vi "main_VI.vi"() -> ()   [LabVIEW 2019]
uses:
  <vilib>/myRIO/Instrument Drivers/Onboard IO/UART/typedef/VISA Configuration.ctl
  <vilib>/Platform/TimedLoop/XDataNode/timing_clust.ctl
  <vilib>/Platform/TimedLoop/XDataNode/nitl_modes.ctl
  <vilib>/Platform/TimedLoop/XDataNode/wakeup.ctl
  <vilib>/myRIO/Instrument Drivers/Onboard IO/AI/typedefs/AI Reference.ctl
  <vilib>/myRIO/Common/Instrument Driver Framework/Utilities/typedefs/myRIO Generic Hardware Reference.ctl
  <vilib>/myRIO/Common/Instrument Driver Framework/Utilities/typedefs/Hardware Version Enum.ctl
  <vilib>/myRIO/Common/Instrument Driver Framework/Utilities/typedefs/myRIO v1.0 Reference.ctl
  <vilib>/myRIO/Common/Instrument Driver Framework/Utilities/typedefs/Generic FPGA Reference.ctl
  <vilib>/myRIO/Common/Instrument Driver Framework/myRIO v1.0/AI/typedefs/AI Channels List.ctl
  <vilib>/myRIO/Common/Instrument Driver Framework/myRIO v1.0/AI/typedefs/AI Channels Enum.ctl
  <vilib>/myRIO/Common/Instrument Driver Framework/Utilities/typedefs/Analog Scaling Constants List.ctl
  <vilib>/myRIO/Common/Instrument Driver Framework/Utilities/typedefs/Analog Scaling Constants.ctl
  <vilib>/userDefined/High Color/nirio_resource_hc.ctl
  <vilib>/Instr/_visa.llb/VISA Configure Serial Port (Instr).vi
  <vilib>/myRIO/Instrument Drivers/Onboard IO/AI/vis/Read.vi
  <vilib>/myRIO/Common/Instrument Driver Framework/myRIO v1.0/AI/vis/myRIO v1.1 Open AI.vi
  <vilib>/myRIO/Common/Instrument Driver Framework/Utilities/vis/Is FPGA Ref Available.vi
  <vilib>/myRIO/Common/Instrument Driver Framework/Utilities/vis/Validate Channels.vi
  <vilib>/myRIO/Common/Instrument Driver Framework/myRIO v1.0/AI/vis/myRIO v1.0 Reserve AI.vi
  <vilib>/myRIO/Common/Instrument Driver Framework/myRIO v1.0/AI/vis/myRIO v1.0 Build MUX Configuration AI.vi
  <vilib>/myRIO/Common/Instrument Driver Framework/myRIO v1.0/Resource Manager/vis/myRIO v1.0 Reserve Channel List.vi
  <vilib>/myRIO/Common/Instrument Driver Framework/myRIO v1.0/Resource Manager/vis/myRIO v1.0 Reserve Channel.vi
  <vilib>/myRIO/Common/Instrument Driver Framework/myRIO v1.0/Resource Manager/vis/myRIO v1.0 Unreserve Channel.vi
  <vilib>/myRIO/Common/Instrument Driver Framework/myRIO v1.0/Resource Manager/vis/myRIO v1.0 Build Mutex Name.vi
  <vilib>/Utility/VariantDataType/GetNumericInfo.vi
  <vilib>/Utility/error.llb/Error Cluster From Error Code.vi
  <vilib>/myRIO/Common/Instrument Driver Framework/myRIO v1.0/myRIO v1.1 Open.vi
  <vilib>/myRIO/Common/Instrument Driver Framework/myRIO v1.0/AI/vis/myRIO v1.0 Get Scaling Constants AI.vi
  <vilib>/myRIO/Common/Instrument Driver Framework/Utilities/vis/IO Manager.vi
  <vilib>/myRIO/Common/Instrument Driver Framework/Utilities/vis/Configuration Manager.vi
  <vilib>/myRIO/Common/Instrument Driver Framework/myRIO v1.0/myRIO v1.0 Close.vi
  <vilib>/myRIO/Common/Instrument Driver Framework/myRIO v1.0/AI/vis/myRIO v1.0 Read AI.vi
  <vilib>/Utility/file.llb/Write Delimited Spreadsheet (DBL).vi
  <vilib>/platform/TimedLoop/XDataNode/XDataNode.xnode
  <vilib>/myRIO/Express VI/Onboard IO/AI/AI Express VI.xnode
  <vilib>/myRIO/Instrument Drivers/Onboard IO/AI/vis/myRIO AI Open.xnode
  <vilib>/Platform/TimedLoop/XDataNode/XDNodeRunTimeDep.lvlib
  <vilib>/myRIO/Instrument Drivers/Onboard IO/UART/UART.lvlib
  <vilib>/myRIO/Instrument Drivers/Onboard IO/AI/AI.lvlib
panel:
  out "# elements 2":u32
  out "element out 2":dbl
  out "# elements":u32
  out "element out":dbl
  out "Gyro_z":dbl
  in  "error in (no error)":errorcluster
  out "On time in":i32
  out "Late in":i32
  out "Loop cycle rate":u32
  in  "File_Num.":i16
  in  "stop":bool
  out "error out":errorcluster
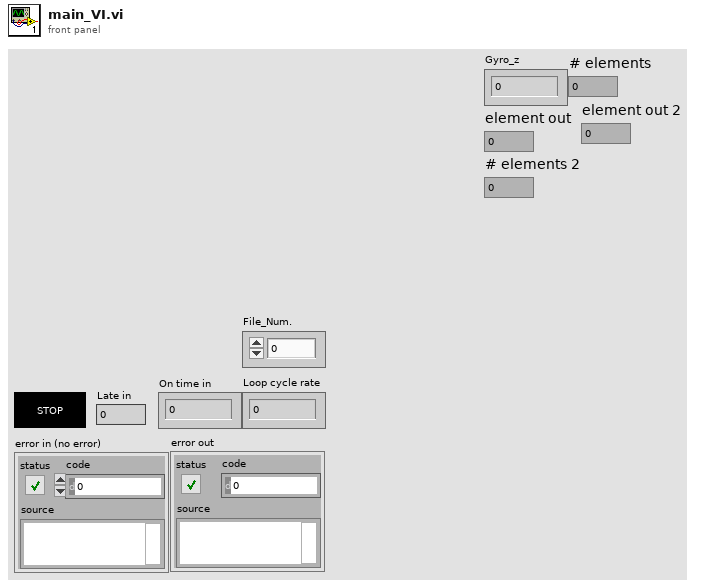
[diagram p1: front panel]
types:
  T1 = cluster{"read mode":enum16{"polling", "blocking"}, "write mode":enum16{"polling", "blocking"}}
  T2 = typedef "UART.lvlib/VISA Configuration.ctl" = cluster{"baud rate (9600)":u32, "data bits (8)":u16, "parity (0:none)":enum16{"None", "Odd", "Even", "Mark", "Space"}, "stop bits (10: 1 bit)":u16, "flow control (0:none)":u16, "termination char\n(0xA = '\\n' = LF) ":u8, "Enable Termination\nChar (T)":bool, "timeout (10sec)":u32}
  T3 = typedef "XDNodeRunTimeDep.lvlib/timing_clust.ctl" = cluster{"Expected End [f-1]":u64, "Actual End [f-1]":u64, "Finished Late? [f-1]":bool, "Expected End [i-1]":u64, "Actual End [i-1]":u64, "Finished Late? [i-1]":bool, "Expected Start [i]":u64, "Actual Start [i]":u64, "Expected Start [f]":u64, "Actual Start [f]":u64, "Source Name":string, "Structure Name":string, "Period":i64, "Deadline":i64, "Offset":i64, "Start":i64, "Priority":i32, "Timeout":i32, "Mode":T4, "Wakeup Reason":T5, "Error":errorcluster, "Source Type":string, "Secondary Source Type":string, "Global End Time":u64, "Global Start Time":u64, "Frame Duration":u64, "Iteration Duration":u64, "Assigned CPU":i32, "I/O Scan Engine Mode":u32}
  T4 = typedef "XDNodeRunTimeDep.lvlib/nitl_modes.ctl" = enum32{"No Change", "Process missed periods, maintain original phase", "Discard missed periods, maintain original phase", "Process missed periods, ignore original phase", "Discard missed periods, ignore original phase"}
  T5 = typedef "XDNodeRunTimeDep.lvlib/wakeup.ctl" = enum32{"Normal", "Aborted", "Asynchronous wakeup", "Timing source error", "Timed loop error", "Timeout"}
  T6 = typedef "AI.lvlib/AI Reference.ctl" = cluster{"myRIO Reference":T7, "AI Channels List":T11, "AI Scaling Constants List":T13}
  T7 = typedef "myRIO Generic Hardware Reference.ctl" = cluster{"myRIO Model":T8, "myRIO Hardware Reference":T9}
  T8 = typedef "Hardware Version Enum.ctl" = enum16{"Unknown", "myRIO-1900", "myRIO-1950", "roboRIO", "NI ELVIS RIO CM", "ELVIS III"}
  T9 = typedef "myRIO v1.0 Reference.ctl" = cluster{"Generic FPGA Reference":T10, "Allow multiple opens":bool}
  T10 = typedef "Generic FPGA Reference.ctl" = refnum<k20>
  T11 = typedef "AI Channels List.ctl" = T12[]
  T12 = typedef "AI Channels Enum.ctl" = enum16{"Not Connected", "AudioIn/Left", "AudioIn/Right", "C/AI0", "C/AI1", "A/AI0", "A/AI1", "A/AI2", "A/AI3", "A/AI4", "A/AI5", "A/AI6", "A/AI7", "B/AI0", "B/AI1", "B/AI2", "B/AI3", "B/AI4", "B/AI5", "B/AI6", "B/AI7", "AI/AI0", "AI/AI1", "AI/AI2", "AI/AI3", "A/AI0 (DIFF)", "A/AI1 (DIFF)", "A/AI2 (DIFF)", "A/AI3 (DIFF)", "B/AI0 (DIFF)", "B/AI1 (DIFF)", "B/AI2 (DIFF)", "B/AI3 (DIFF)"}
  T13 = typedef "Analog Scaling Constants List.ctl" = T14[]
  T14 = typedef "Analog Scaling Constants.ctl" = cluster{"LSB Weight (Volts)":dbl, "Offset (Volts)":dbl, "Signed?":bool}
  T15 = typedef "nirio_resource_hc.ctl" = tag
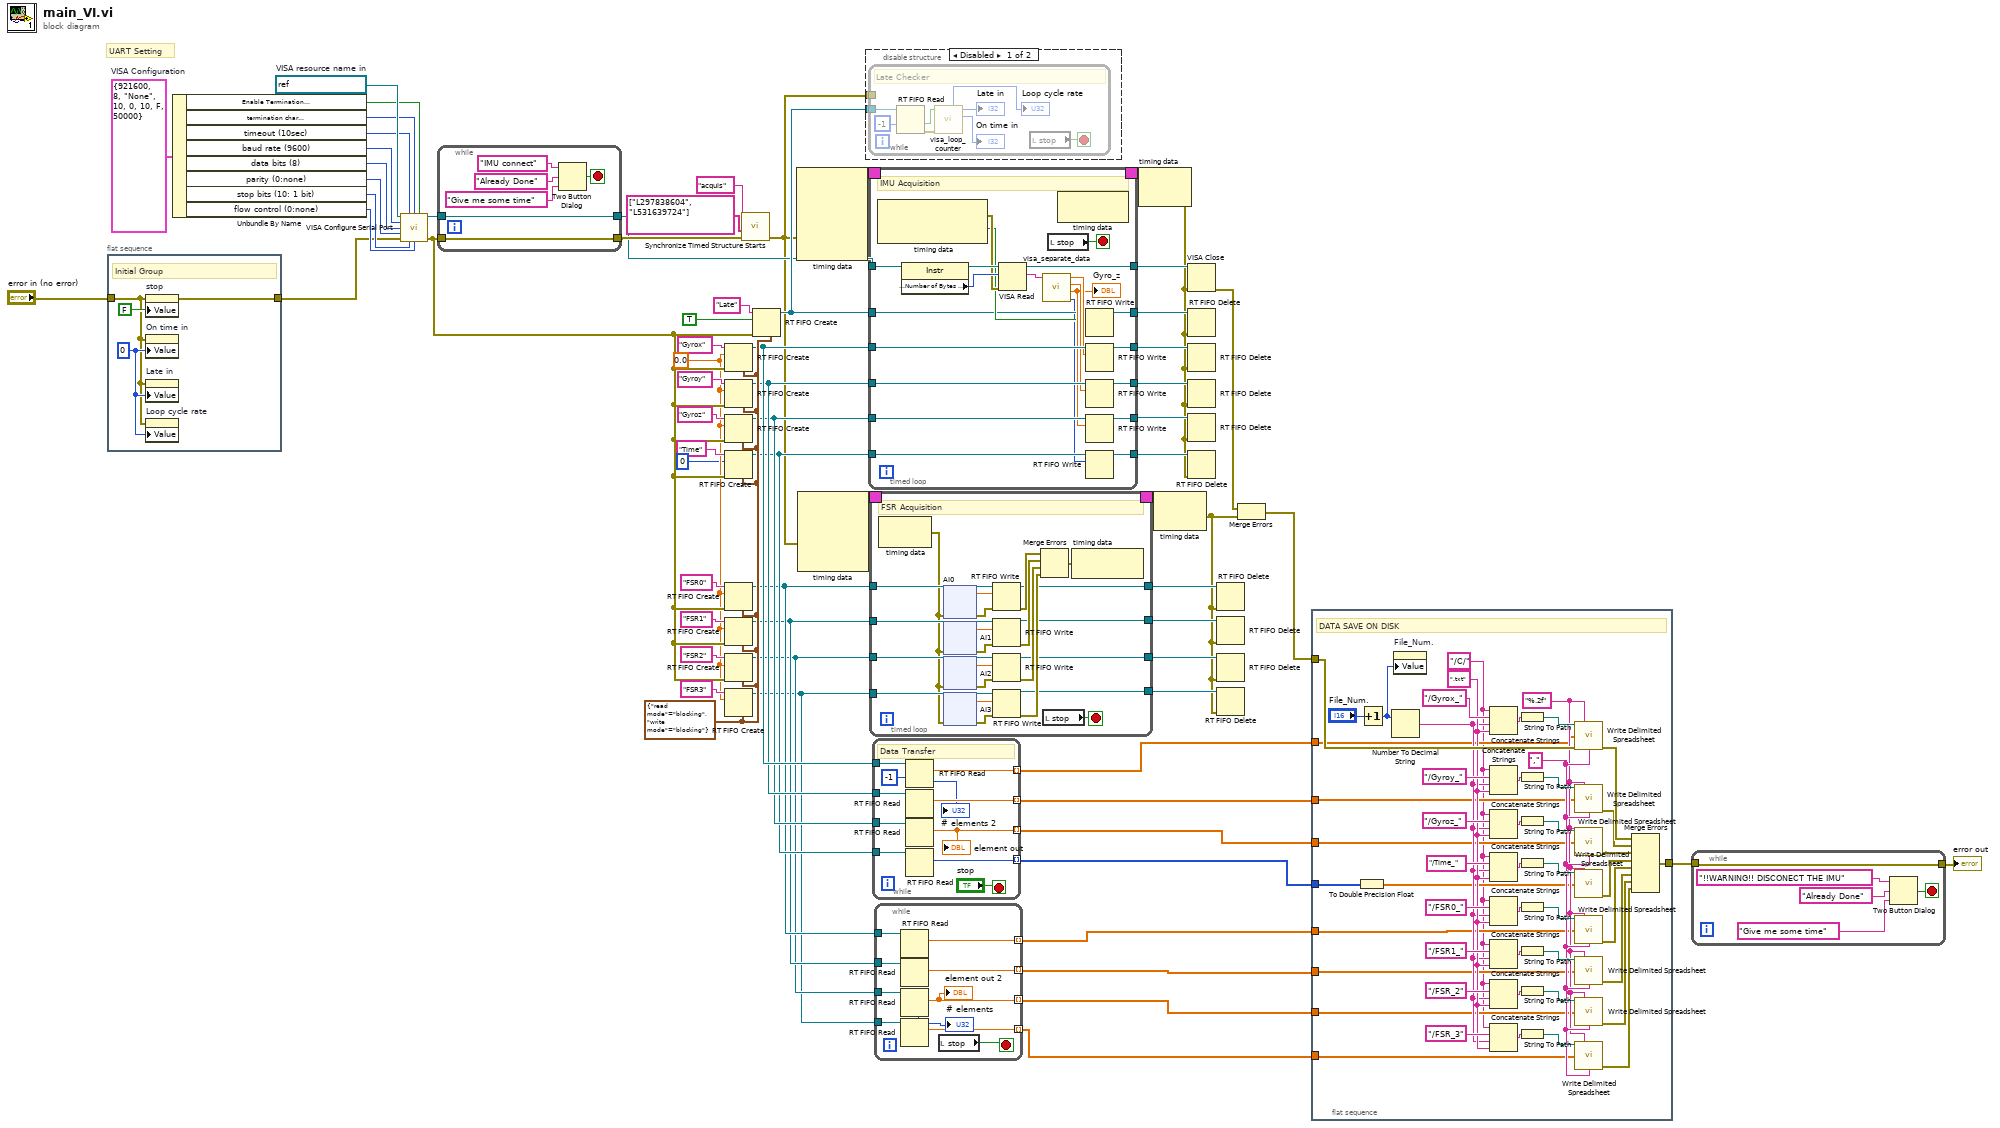
[diagram p0: block diagram]
diagram:
  w43 = T1 {"read mode"=enum."blocking", "write mode"=enum."blocking"} ("r/w modes (polling,polling)")
  w42 = 0.0
  w66 = T2 {"baud rate (9600)"=921600, "data bits (8)"=8, "parity (0:none)"=enum."None", "stop bits (10: 1 bit)"=10, "flow control (0:none)"=0, "termination char\n(0xA = '\\n' = LF) "=10, "Enable Termination\nChar (T)"=FALSE, "timeout (10sec)"=50000}  # VISA Configuration
  w67 = refnum<visa-resource-name> "ASRL1::INSTR"  # VISA resource name in
  # "UART Setting"
  n1 = flat-sequence {
    tunnel: "error in (no error)" -> [w71]
    tunnel: [w70] -> w23
    frame #0 {
      w72 = u16 0 ("On time in")
      # "Initial Group"
      n2 = property on="stop" class="Bool (strict)"(error in=w71, "Value"=FALSE ("stop")) -> (error out=w70:errorcluster)  [unwired: 1 in, 1 out]
      n3 = property on="On time in" class="DigNum (strict)"(error in=w71, "Value"=w72) -> ()  [unwired: 1 in, 2 out]
      n4 = property on="Late in" class="DigNum (strict)"(error in=w71, "Value"=w72) -> ()  [unwired: 1 in, 2 out]
      n5 = property on="Loop cycle rate" class="DigNum (strict)"(error in=w71, "Value"=w72) -> ()  [unwired: 1 in, 2 out]
    }
  }
  n6 = Unbundle By Name(w66) -> ("Enable Termination\nChar (T)"=w65:bool, "termination char\n(0xA = '\\n' = LF)"=w64:u8, "timeout (10sec)"=w63:u32, "baud rate (9600)"=w59:u32, "data bits (8)"=w60:u16, "parity (0:none)"=w61:enum16{"None", "Odd", "Even", "Mark", "Space"}, "stop bits (10: 1 bit)"=w62:u16, "flow control (0:none)"=w58:u16)
  n7 = call-poly "VISA Configure Serial Port"("VISA resource name"=w67, "timeout (10sec)"=w63, "termination char\n(0xA = '\\n' = LF)"=w64, "Enable Termination\nChar (T)"=w65, "baud rate (9600)"=w59, "data bits (8)"=w60, "parity (0:none)"=w61, "error in (no error)"=w23, "stop bits (10: 1 bit)"=w62, "flow control (0:none)"=w58) -> ("VISA resource name out"=w55:refnum<visa-resource-name>, "error out"=w45:errorcluster)  [unwired: 4 in]
  n8 = while {
    tunnel: [w79] -> w35
    tunnel: w45 -> [w79]
    tunnel: [w78] -> w34
    tunnel: w55 -> [w78]
    stop <- w74 stop-if-true
    n9 = Two Button Dialog(message="IMU connect", 1:"Give me some time" ("F button name (\"Cancel\")"), 2:"Already Done" ("button name (\"OK\")")) -> (T button?=w74:bool)
  }
  n10 = RT FIFO Create(0:"Gyrox" ("name (unnamed)"), 1:w42, 3:w45, 7:w43) -> (8:w33:refnum<k33>)  [unwired: 4 in, 2 out]
  n11 = RT FIFO Create(0:"Gyroy" ("name (unnamed)"), 1:w42, 3:w45, 7:w43) -> (8:w32:refnum<k33>)  [unwired: 4 in, 2 out]
  n12 = RT FIFO Create(0:"Gyroz" ("name (unnamed)"), 1:w42, 3:w45, 7:w43) -> (8:w31:refnum<k33>)  [unwired: 4 in, 2 out]
  n13 = RT FIFO Create(0:"Time" ("name (unnamed)"), 1:0 ("Time"), 3:w45, 7:w43) -> (8:w30:refnum<k33>)  [unwired: 4 in, 2 out]
  n14 = RT FIFO Create(0:"FSR0" ("name (unnamed)"), 1:w42, 3:w45, 7:w43) -> (8:w8:refnum<k33>)  [unwired: 4 in, 2 out]
  n15 = RT FIFO Create(0:"FSR1" ("name (unnamed)"), 1:w42, 3:w45, 7:w43) -> (8:w7:refnum<k33>)  [unwired: 4 in, 2 out]
  n16 = RT FIFO Create(0:"FSR2" ("name (unnamed)"), 1:w42, 3:w45, 7:w43) -> (8:w6:refnum<k33>)  [unwired: 4 in, 2 out]
  n17 = RT FIFO Create(0:"FSR3" ("name (unnamed)"), 1:w42, 7:w43) -> (8:w5:refnum<k33>)  [unwired: 5 in, 2 out]
  n18 = call <vilib>:"Synchronize Timed Structure Starts.vi"("error in (no error)"=w35, "timed structure names"=string[] ["L297838604", "L531639724"], "synchronization group name"="acquis") -> ("error out"=w22:errorcluster)  [unwired: 7 in, 1 out]
  n19 = RT FIFO Create(0:"Late" ("name (unnamed)"), 1:TRUE, 3:w45, 7:w43) -> (8:w40:refnum<k33>)  [unwired: 4 in, 2 out]
  n20 = node-c288(w22) -> (w69:T3)  [unwired: 4 in]
  n21 = node-c288(w22) -> (w39:T3)  [unwired: 3 in]
  n22 = disable-structure shown="Disabled" {
    disable-tunnel: w40 -> [w81 _]
    disable-tunnel: w22 -> [w80 _]
    frame Disabled {
      n23 = while {
        tunnel: w81 -> [w83]
        tunnel: w80 -> [_]
        stop <- w84 stop-if-true
        # "Late Checker"
        n24 = RT FIFO Read(0:w83, 2:-1 ("timeout in ms (0)")) -> (10:w86:bool, 11:w85:errorcluster)  [unwired: 2 in, 3 out]
        n25 = call "visa_loop_counter.vi"("Error In"=w85, "Finished Late? [i-1]"=w86) -> ("On time counter buffer in"=→"On time in":i32, "Late counter buffer in"=→"Late in":i32, "Loop cycle rate"=→"Loop cycle rate":u32)  [unwired: 5 in, 2 out]
        n26 = local read "stop"() -> (w84:bool)
      }
    }
    frame Enabled {
    }
  }
  n27 = timed-loop {
    timing: w69 -> [_]
    timing-out: [_] -> w68
    tunnel: w33 -> [w105]
    tunnel: w32 -> [w104]
    tunnel: w31 -> [w103]
    tunnel: [w102] -> w20
    tunnel: [w101] -> w19
    tunnel: [w100] -> w17
    tunnel: w40 -> [w95]
    tunnel: [w94] -> w21
    tunnel: w30 -> [w93]
    tunnel: [w91] -> w18
    tunnel: w34 -> [w109]
    tunnel: [w108] -> w57
    stop <- w90 stop-if-true
    # "IMU Acquisition"
    n28 = node-c288() -> (w107:errorcluster, w96:bool)  [unwired: 1 in]
    n29 = property class="Instr"(reference=w109) -> (reference out=w111:refnum<visa-resource-name>, "Serial Settings:Number of Bytes at Serial Port"=w110:u32)  [unwired: 1 in, 1 out]
    n30 = VISA Read(VISA resource name=w111, byte count=w110, error in (no error)=w107) -> (VISA resource name out=w108:refnum<visa-resource-name>, read buffer=w106:string)  [unwired: 2 out]
    n31 = call "visa_separate_data.vi"("Input string"=w106) -> ("Time"=w92:i32, "Gyro_z"=w97:dbl, "Gyro_y"=w98:dbl, "Gyro_x"=w99:dbl)  [unwired: 7 in]
    "Gyro_z" <- w97
    n32 = local read "stop"() -> (w90:bool)
    n33 = node-c288() -> ()  [unwired: 1 in, 1 out]
    n34 = RT FIFO Write(0:w95, 1:w96) -> (8:w94:refnum<k33>)  [unwired: 3 in, 3 out]
    n35 = RT FIFO Write(0:w105, 1:w99) -> (8:w102:refnum<k33>)  [unwired: 3 in, 3 out]
    n36 = RT FIFO Write(0:w104, 1:w98) -> (8:w101:refnum<k33>)  [unwired: 3 in, 3 out]
    n37 = RT FIFO Write(0:w103, 1:w97) -> (8:w100:refnum<k33>)  [unwired: 3 in, 3 out]
    n38 = RT FIFO Write(0:w93, 1:w92) -> (8:w91:refnum<k33>)  [unwired: 3 in, 3 out]
  }
  n39 = timed-loop {
    timing: w39 -> [_]
    timing-out: [_] -> w38
    tunnel: w8 -> [w138]
    tunnel: w7 -> [w137]
    tunnel: w6 -> [w136]
    tunnel: w5 -> [w135]
    tunnel: [w119] -> w15
    tunnel: [w118] -> w14
    tunnel: [w117] -> w13
    tunnel: [w116] -> w12
    stop <- w134 stop-if-true
    # "FSR Acquisition"
    n40 = node-c288() -> (w129:errorcluster)  [unwired: 1 in]
    n41 = xnode ("AI0")("error in (no error)"=w129) -> ("error out"=w125:errorcluster, "A/AI0 (Pin 3)"=w133:dbl)
    n42 = xnode ("AI1")("error in (no error)"=w129) -> ("error out"=w126:errorcluster, "A/AI1 (Pin 5)"=w132:dbl)
    n43 = xnode ("AI2")("error in (no error)"=w129) -> ("error out"=w127:errorcluster, "A/AI2 (Pin 7)"=w131:dbl)
    n44 = xnode ("AI3")("error in (no error)"=w129) -> ("error out"=w128:errorcluster, "A/AI3 (Pin 9)"=w130:dbl)
    n45 = RT FIFO Write(0:w138, 1:w133, 3:w125) -> (8:w119:refnum<k33>, 11:w121:errorcluster)  [unwired: 2 in, 2 out]
    n46 = RT FIFO Write(0:w137, 1:w132, 3:w126) -> (8:w118:refnum<k33>, 11:w122:errorcluster)  [unwired: 2 in, 2 out]
    n47 = RT FIFO Write(0:w136, 1:w131, 3:w127) -> (8:w117:refnum<k33>, 11:w123:errorcluster)  [unwired: 2 in, 2 out]
    n48 = RT FIFO Write(0:w135, 1:w130, 3:w128) -> (8:w116:refnum<k33>, 11:w124:errorcluster)  [unwired: 2 in, 2 out]
    n49 = Merge Errors(w121, w122, w123, w124) -> (w120:errorcluster)
    n50 = local read "stop"() -> (w134:bool)
    n51 = node-c288(w120) -> ()  [unwired: 1 out]
  }
  n52 = while {
    tunnel: w33 -> [w302]
    tunnel: w32 -> [w301]
    tunnel: w31 -> [w300]
    tunnel: w30 -> [w299]
    tunnel: [w298] -> w29 mode=indexing
    tunnel: [w297] -> w28 mode=indexing
    tunnel: [w296] -> w27 mode=indexing
    tunnel: [w295] -> w26 mode=indexing
    stop <- "stop" stop-if-true
    # "Data Transfer"
    n53 = RT FIFO Read(0:w302, 2:-1 ("timeout in ms (0)")) -> (7:→"# elements 2":u32, 9:w298:dbl)  [unwired: 2 in, 3 out]
    n54 = RT FIFO Read(0:w301) -> (9:w297:dbl)  [unwired: 3 in, 4 out]
    n55 = RT FIFO Read(0:w300) -> (9:w296:dbl)  [unwired: 3 in, 4 out]
    "element out" <- w296
    n56 = RT FIFO Read(0:w299) -> (9:w295:i32)  [unwired: 3 in, 4 out]
  }
  n57 = while {
    tunnel: w8 -> [w312]
    tunnel: w7 -> [w311]
    tunnel: w6 -> [w310]
    tunnel: w5 -> [w309]
    tunnel: [w308] -> w4 mode=indexing
    tunnel: [w307] -> w3 mode=indexing
    tunnel: [w305] -> w2 mode=indexing
    tunnel: [w306] -> w1 mode=indexing
    stop <- w303 stop-if-true
    n58 = RT FIFO Read(0:w312) -> (9:w308:dbl)  [unwired: 3 in, 4 out]
    n59 = RT FIFO Read(0:w311) -> (9:w306:dbl)  [unwired: 3 in, 4 out]
    n60 = RT FIFO Read(0:w310) -> (7:→"# elements":u32, 9:w305:dbl)  [unwired: 3 in, 3 out]
    "element out 2" <- w305
    n61 = RT FIFO Read(0:w309) -> (9:w307:dbl)  [unwired: 3 in, 4 out]
    n62 = local read "stop"() -> (w303:bool)
  }
  n63 = node-c288(w68) -> (w16:errorcluster)
  n64 = node-c288(w38) -> (w11:errorcluster)
  n65 = VISA Close(VISA resource name=w57, error in (no error)=w16) -> (error out=w25:errorcluster)
  n66 = RT FIFO Delete(0:w21, 3:w16) -> ()  [unwired: 1 in, 1 out]
  n67 = RT FIFO Delete(0:w20, 3:w16) -> ()  [unwired: 1 in, 1 out]
  n68 = RT FIFO Delete(0:w19, 3:w16) -> ()  [unwired: 1 in, 1 out]
  n69 = RT FIFO Delete(0:w17, 3:w16) -> ()  [unwired: 1 in, 1 out]
  n70 = RT FIFO Delete(0:w18, 3:w16) -> ()  [unwired: 1 in, 1 out]
  n71 = RT FIFO Delete(0:w15, 3:w11) -> ()  [unwired: 1 in, 1 out]
  n72 = RT FIFO Delete(0:w14, 3:w11) -> ()  [unwired: 1 in, 1 out]
  n73 = RT FIFO Delete(0:w13, 3:w11) -> ()  [unwired: 1 in, 1 out]
  n74 = RT FIFO Delete(0:w12, 3:w11) -> ()  [unwired: 1 in, 1 out]
  n75 = Merge Errors(w25, w11) -> (w10:errorcluster)
  n76 = flat-sequence {
    tunnel: w10 -> [w359]
    tunnel: [w316] -> w9
    tunnel: w28 -> [w331]
    tunnel: w27 -> [w330]
    tunnel: w26 -> [w315]
    tunnel: w4 -> [w329]
    tunnel: w1 -> [w328]
    tunnel: w2 -> [w327]
    tunnel: w3 -> [w326]
    tunnel: w29 -> [w325]
    frame #0 {
      w334 = ".txt" ("string")
      w313 = "/C/" ("string")
      w335 = "," ("delimiter (\\t)")
      w332 = "%.2f" ("format (%.3f)")
      # "DATA SAVE ON DISK"
      n77 = To Double Precision Float(number=w315) -> (double precision float=w314:dbl[])
      n78 = Increment(x="File_Num.") -> (x+1=w358:i16)
      n79 = Number To Decimal String(number=w358) -> (decimal integer string=w333:string)  [unwired: 1 in]
      n80 = property on="File_Num." class="DigNum (strict)"("Value"=w358) -> ()  [unwired: 2 in, 2 out]
      n81 = Concatenate Strings(w313, "/Gyrox_" ("string"), w333, w334) -> (w362:string)
      n82 = Concatenate Strings(w313, "/Gyroy_" ("string"), w333, w334) -> (w355:string)
      n83 = Concatenate Strings(w313, "/Gyroz_" ("string"), w333, w334) -> (w352:string)
      n84 = Concatenate Strings(w313, "/Time_" ("string"), w333, w334) -> (w349:string)
      n85 = Concatenate Strings(w313, "/FSR0_" ("string"), w333, w334) -> (w346:string)
      n86 = Concatenate Strings(w313, "/FSR1_" ("string"), w333, w334) -> (w343:string)
      n87 = Concatenate Strings(w313, "/FSR_2" ("string"), w333, w334) -> (w340:string)
      n88 = Concatenate Strings(w313, "/FSR_3" ("string"), w333, w334) -> (w337:string)
      n89 = String To Path(string=w362) -> (path=w361:path)
      n90 = String To Path(string=w355) -> (path=w356:path)
      n91 = String To Path(string=w352) -> (path=w351:path)
      n92 = String To Path(string=w349) -> (path=w350:path)
      n93 = String To Path(string=w346) -> (path=w345:path)
      n94 = String To Path(string=w343) -> (path=w344:path)
      n95 = String To Path(string=w340) -> (path=w339:path)
      n96 = String To Path(string=w337) -> (path=w338:path)
      n97 = call-poly <vilib>:"Write Delimited Spreadsheet.vi"("file path (dialog if empty)"=w361, "format (%.3f)"=w332, "1D data"=w325, "error in (no error)"=w359, "delimiter (\\t)"=w335) -> ("error out"=w324:errorcluster)  [unwired: 9 in, 1 out]
      n98 = call-poly <vilib>:"Write Delimited Spreadsheet.vi"("file path (dialog if empty)"=w356, "format (%.3f)"=w332, "1D data"=w331, "delimiter (\\t)"=w335) -> ("error out"=w323:errorcluster)  [unwired: 10 in, 1 out]
      n99 = call-poly <vilib>:"Write Delimited Spreadsheet.vi"("file path (dialog if empty)"=w351, "format (%.3f)"=w332, "1D data"=w330, "delimiter (\\t)"=w335) -> ("error out"=w322:errorcluster)  [unwired: 10 in, 1 out]
      n100 = call-poly <vilib>:"Write Delimited Spreadsheet.vi"("file path (dialog if empty)"=w350, "format (%.3f)"=w332, "1D data"=w314) -> ("error out"=w321:errorcluster)  [unwired: 11 in, 1 out]
      n101 = call-poly <vilib>:"Write Delimited Spreadsheet.vi"("file path (dialog if empty)"=w345, "format (%.3f)"=w332, "1D data"=w329, "delimiter (\\t)"=w335) -> ("error out"=w320:errorcluster)  [unwired: 10 in, 1 out]
      n102 = call-poly <vilib>:"Write Delimited Spreadsheet.vi"("file path (dialog if empty)"=w344, "format (%.3f)"=w332, "1D data"=w328, "delimiter (\\t)"=w335) -> ("error out"=w319:errorcluster)  [unwired: 10 in, 1 out]
      n103 = call-poly <vilib>:"Write Delimited Spreadsheet.vi"("file path (dialog if empty)"=w339, "format (%.3f)"=w332, "1D data"=w327, "delimiter (\\t)"=w335) -> ("error out"=w318:errorcluster)  [unwired: 10 in, 1 out]
      n104 = call-poly <vilib>:"Write Delimited Spreadsheet.vi"("file path (dialog if empty)"=w338, "format (%.3f)"=w332, "1D data"=w326, "delimiter (\\t)"=w335) -> ("error out"=w317:errorcluster)  [unwired: 10 in, 1 out]
      n105 = Merge Errors(w324, w323, w322, w321, w320, w319, w318, w317) -> (w316:errorcluster)
    }
  }
  n106 = while {
    tunnel: [w367] -> w56
    tunnel: w9 -> [w367]
    stop <- w363 stop-if-true
    n107 = Two Button Dialog(message="!!WARNING!! DISCONECT THE IMU", 1:"Give me some time" ("F button name (\"Cancel\")"), 2:"Already Done" ("button name (\"OK\")")) -> (T button?=w363:bool)
  }
  "error out" <- w56
